vi "AFG3352X.set SWIFT.vi"(0 "i ref in":refnum<vi>, 1 "Amplitude (0.1 Vpp)":dbl=0.1, 2 "Offset (0 V)":dbl, 3 "Sample Rate (40000 Sa/s)":dbl=40000.0, 4 "Apodized SWIFT":dbl[](array[numeric])=array[65000 elements], 5 "error in (no error)":errorcluster) -> (14 "i ref out":refnum<vi>, 19 "error out":errorcluster)   [LabVIEW 2014, in "AFG3352X.lvlib"]
doc: "Set function for SWIFT operation. This will already switches on the output."
uses:
  AFG3352X.lvlib
  instr.lib/Agilent 3352X Series/Agilent 3352X Series.lvlib
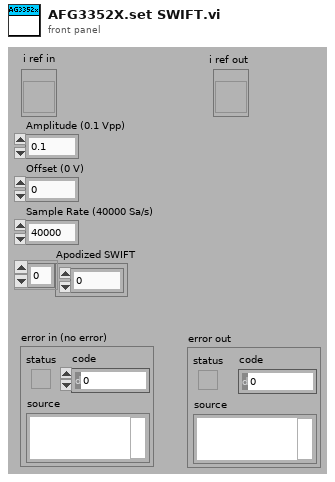
[diagram p1: front panel]
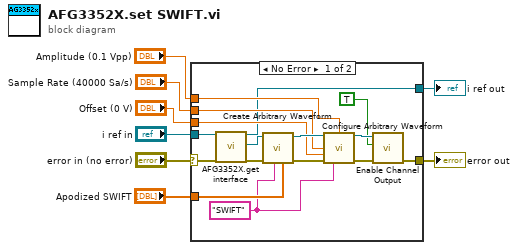
[diagram p0: block diagram]
diagram:
  n1 = case shown="No Error" "error in (no error)" {
    selector: "error in (no error)" -> [w12 w26]
    tunnel: [w14 w26] -> w8
    tunnel: "Apodized SWIFT" -> [w24 _]
    tunnel: "Sample Rate (40000 Sa/s)" -> [w21 _]
    tunnel: "Offset (0 V)" -> [w20 _]
    tunnel: "Amplitude (0.1 Vpp)" -> [w18 _]
    tunnel: "i ref in" -> [w13 w25]
    tunnel: [w11 w25] -> w1
    frame No Error {
      w19 = "SWIFT" ("Arbitrary Waveform Name (ARB1)")
      n2 = call "AFG3352X.get interface.vi"("i ref in"=w13, "error in (no error)"=w12) -> ("i ref out"=w11:refnum<vi>, "interface"=w9:refnum<visa-resource-name>, "error out"=w10:errorcluster)  [unwired: 15 in]
      n3 = call "Create Arbitrary Waveform.vi"("Arbitrary Waveform Data"=w24, "Arbitrary Waveform Name (ARB1)"=w19, "error in (no error)"=w10, "VISA resource name"=w9) -> ("error out"=w22:errorcluster, "VISA resource name out"=w23:refnum<visa-resource-name>)  [unwired: 6 in]
      n4 = call "Configure Arbitrary Waveform.vi"("VISA resource name"=w23, "Amplitude (0.1 Vpp)"=w18, "Sample Rate (40000 Sa/s)"=w21, "Offset (0 V)"=w20, "error in (no error)"=w22, "Arbitrary Waveform (ARB1)"=w19) -> ("VISA resource name out"=w17:refnum<visa-resource-name>, "error out"=w16:errorcluster)  [unwired: 8 in]
      n5 = call "Enable Channel Output.vi"("error in (no error)"=w16, "Enable Output (T: Enable)"=TRUE, "VISA resource name"=w17) -> ("error out"=w14:errorcluster)  [unwired: 7 in, 1 out]
    }
    frame Error {
    }
  }
  "error out" <- w8
  "i ref out" <- w1
